vi "Read AI Data.vi"(8 "error in (no error)":errorcluster, 11 "BNT_DAQmx-MCSV-Data in":refnum<class "BNT_DAQmx-MCSV-Data.lvclass">) -> (0 "error out":errorcluster, 2 "AI Data":dbl[](array[numeric]), 3 "BNT_DAQmx-MCSV-Data out":refnum<class "BNT_DAQmx-MCSV-Data.lvclass">)   [LabVIEW 2020, in "BNT_DAQmx.lvlib" / "BNT_DAQmx-MCSV-Data.lvclass"]
doc: "Read AI data."
uses:
  BNT_DAQmx-MCSV-Data.lvclass
  BNT_DAQmx-MCSV-Data.lvclass/BNT_DAQmx-MCSV-Data.ctl
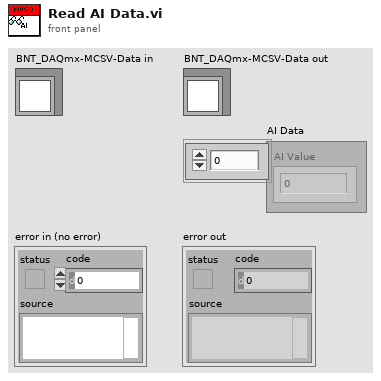
[diagram p1: front panel]
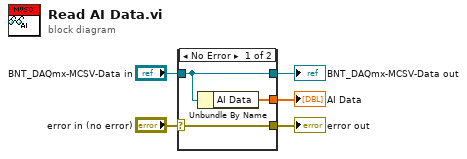
[diagram p0: block diagram]
diagram:
  n1 = case shown="No Error" "error in (no error)" {
    selector: "error in (no error)" -> [w8 w9]
    tunnel: [w8 w9] -> w4
    tunnel: [w7 w10] -> w2
    tunnel: "BNT_DAQmx-MCSV-Data in" -> [w7 w10]
    tunnel: [w6 _] -> w1
    frame No Error {
      n2 = Unbundle By Name(w7) -> ("AI Data"=w6:dbl[])
    }
    frame Error {
    }
  }
  "error out" <- w4
  "BNT_DAQmx-MCSV-Data out" <- w2
  "AI Data" <- w1
